vi "ArmControlManual.vi"(5 "Override Height Limit":bool, 6 "Wrist PID?":bool, 7 "Extension Triggers":cluster{"Retract":dbl, "Extend":dbl}, 8 "error in (no error)":errorcluster, 9 "Pivot Stick":cluster{"X":dbl, "Y":dbl}, 10 "Wrist Stick":cluster{"X":dbl, "Y":dbl}, 11 "Pivot Multiplier":dbl=0.75) -> (0 "error out":errorcluster)   [LabVIEW 2015]
uses:
  <vilib>/Rock Robotics/WPI/CAN/TalonSRX/WPI_CANTalonSRX_APIControlMode.ctl
  Robot Global Data.vi
panel:
  in  "Retract Multiplier":dbl=0.6
  in  "Wrist Multiplier":dbl=45.0 format="%#_13g"
  in  "Extend Multiplier":dbl=1.0
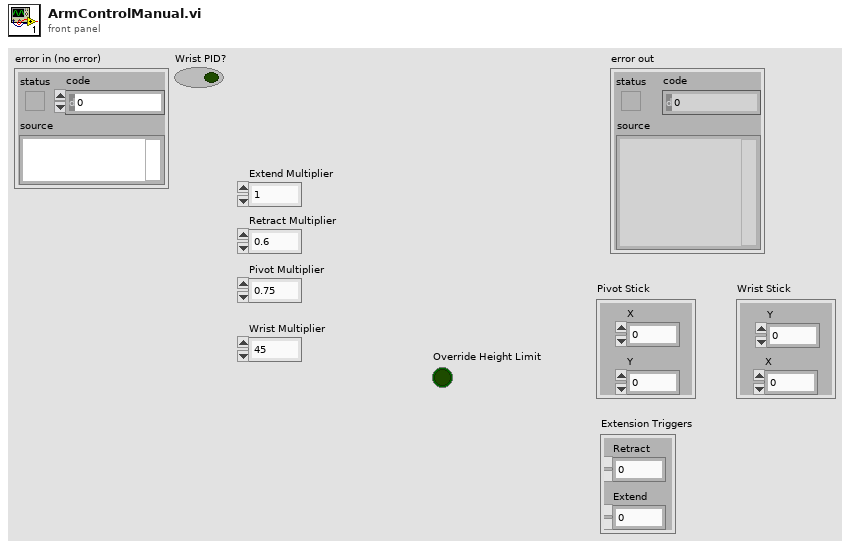
[diagram p1: front panel]
types:
  T1 = typedef "WPI_MotorControlDeviceRef.ctl" = cluster{"DeviceStatus":errorcluster, "Type":T2, "PWM":cluster{"PWM Channel":T3, "DeadBand":T4}, "CAN":cluster{"Device Number":u8, "Control Mode":T5, "Semaphore":T6, "Max Vout":dbl, "TalonSRX Control Mode":T7}, "Invert":bool, "TransformRef":T8, "InvTransformRef":T8}
  T2 = typedef "WPI_MotorControlType.ctl" = enum16{"PWM", "CAN", "CANTalonSRX"}
  T3 = typedef "FPGA_DIOPWMChannel.ctl" = enum8{"PWM 0", "PWM 1", "PWM 2", "PWM 3", "PWM 4", "PWM 5", "PWM 6", "PWM 7", "PWM 8", "PWM 9", "PWM MXP 0", "PWM MXP 1", "PWM MXP 2", "PWM MXP 3", "PWM MXP 4", "PWM MXP 5", "PWM MXP 6", "PWM MXP 7", "PWM MXP 8", "PWM MXP 9", "Invalid"}
  T4 = typedef "WPI_PWMDeadband.ctl" = cluster{"Name":string, "maxPositivePwm":i32, "minPositivePwm":i32, "centerPwm":i32, "maxNegativePwm":i32, "minNegativePwm":i32, "angularRange":u16}
  T5 = typedef "WPI_CANJaguar_ControlMode.ctl" = enum8{"Percent VBus", "Current", "Speed", "Position", "Voltage"}
  T6 = typedef "Semaphore RefNum" = refnum<k1>
  T7 = typedef "WPI_CANTalonSRX_APIControlMode.ctl" = enum8{"Percent VBus", "Speed", "Position", "Slave", "Unchanged / Invalid"}
  T8 = typedef "WPI_PWMTransform_ConPane.ctl" = refnum<vi>
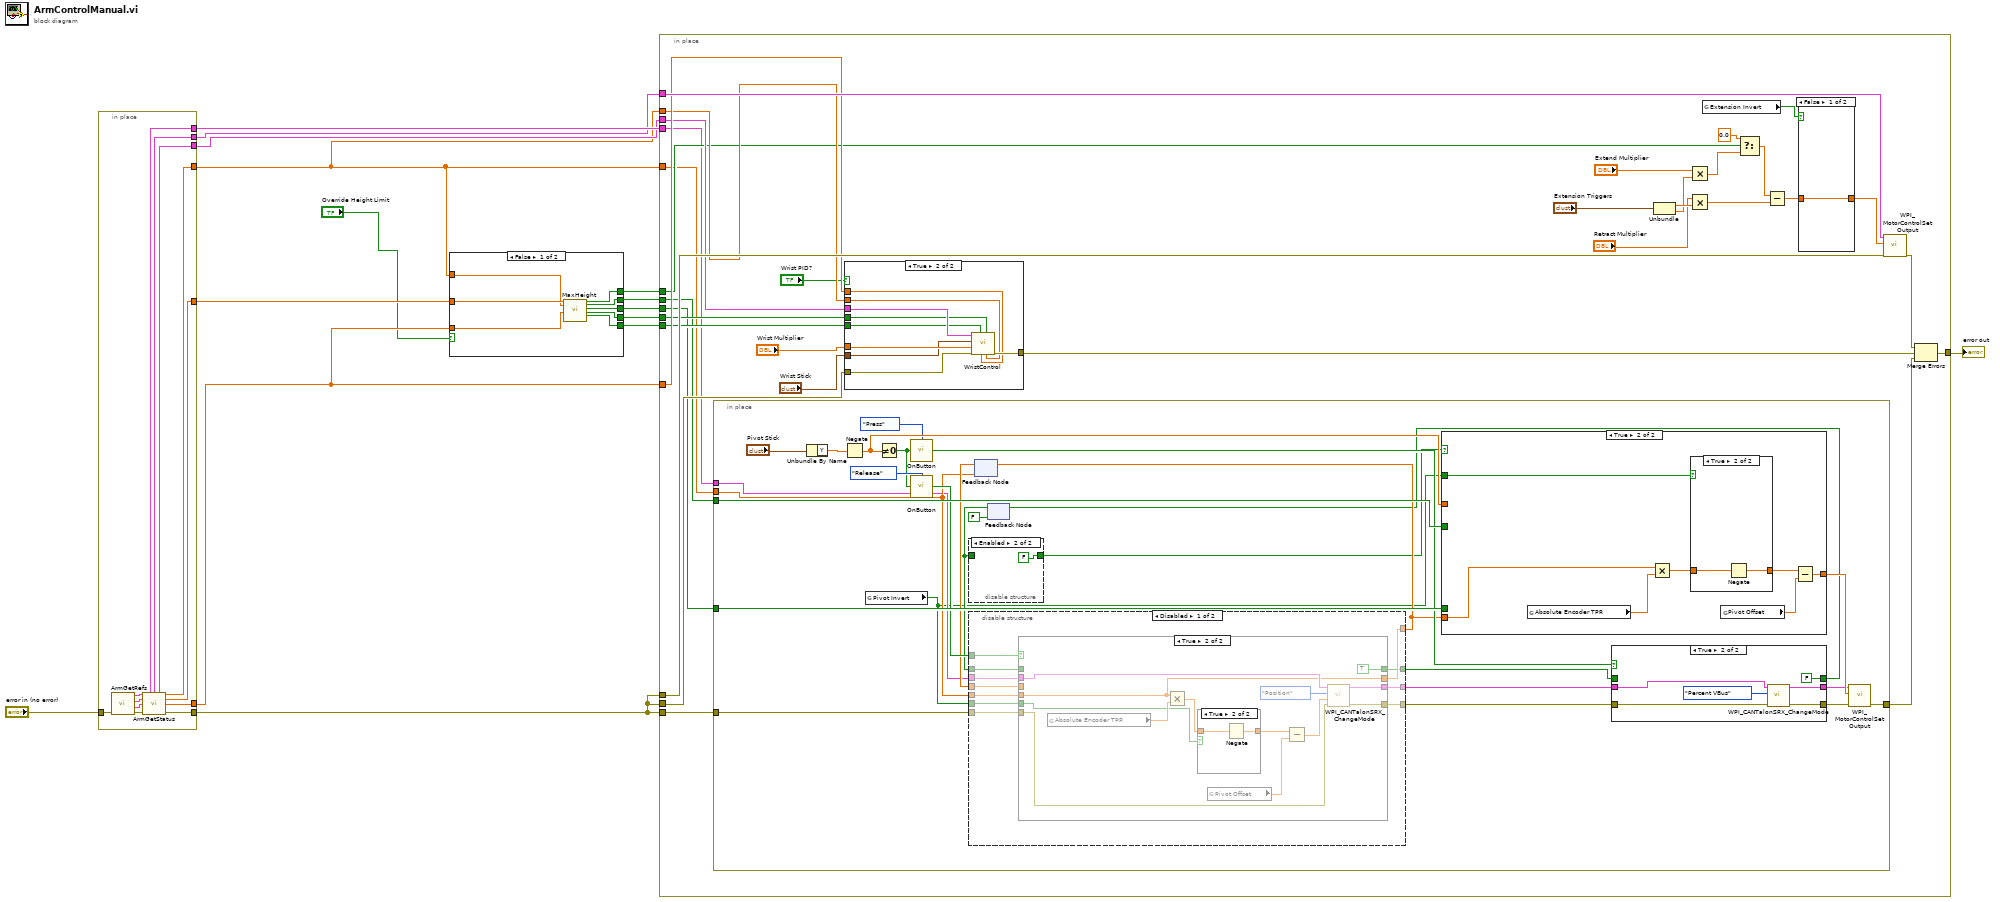
[diagram p0: block diagram]
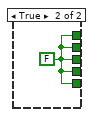
[diagram p2: hidden frame]
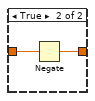
[diagram p3: hidden frame]
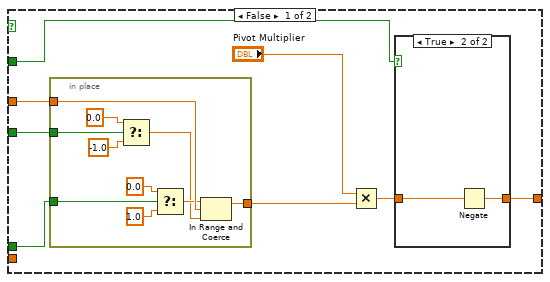
[diagram p9: hidden frame]
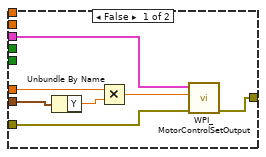
[diagram p12: hidden frame]
diagram:
  n1 = in-place {
    in-place-border: "error in (no error)" -> [w17]
    in-place-border: [w23] -> w14
    in-place-border: [w19] -> w10
    in-place-border: [w22] -> w8
    in-place-border: [w18] -> w12
    in-place-border: [w20] -> w2
    in-place-border: [w16] -> w11
    in-place-border: [w21] -> w9
    n2 = call "ArmGetRefs.vi"("error in (no error)"=w17) -> ("error out"=w24:errorcluster, "Wrist Ref"=w25:T1, "Extension Ref"=w26:T1, "Pivot Ref"=w27:T1)  [unwired: 7 in]
    n3 = call "ArmGetStatus.vi"("Pivot Ref"=w27, "ExtensionRef"=w26, "Wrist Ref"=w25, "error in (no error)"=w24) -> ("Pivot Ref out"=w18:T1, "Extension Ref out"=w19:T1, "Wrist Ref out"=w16:T1, "Pivot angle (rad)"=w20:dbl, "Extension (in.)"=w23:dbl, "Wrist angle (rad, relative to ground)"=w21:dbl, "error out"=w22:errorcluster)  [unwired: 3 in, 2 out]
  }
  n4 = case shown="False" "Override Height Limit" {
    tunnel: w14 -> [w35 _]
    tunnel: w9 -> [w34 _]
    tunnel: [w33 w36] -> w7
    tunnel: [w32 w36] -> w6
    tunnel: [w31 w36] -> w5
    tunnel: [w30 w36] -> w4
    tunnel: [w29 w36] -> w3
    tunnel: w2 -> [w28 _]
    frame False {
      n5 = call "MaxHeight.vi"("Extension Length"=w35, "Pivot Angle"=w28, "Wrist Angle (relative to ground)"=w34) -> ("Disable Extend"=w29:bool, "Disable Pivot Reverse"=w30:bool, "Disable Pivot Forward"=w31:bool, "Disable Wrist Reverse"=w33:bool, "Disable Wrist Forward"=w32:bool)  [unwired: 10 in, 2 out]
    }
    frame True {
      w36 = FALSE
    }
  }
  n6 = in-place {
    in-place-border: [w67] -> w15
    in-place-border: w12 -> [w39]
    in-place-border: w11 -> [w52]
    in-place-border: w10 -> [w61]
    in-place-border: w8 -> [w55]
    in-place-border: w9 -> [w54]
    in-place-border: w2 -> [w53]
    in-place-border: w8 -> [w51]
    in-place-border: w8 -> [w38]
    in-place-border: w7 -> [w45]
    in-place-border: w6 -> [w44]
    in-place-border: w5 -> [w43]
    in-place-border: w4 -> [w42]
    in-place-border: w3 -> [w41]
    in-place-border: w2 -> [w40]
    n7 = in-place {
      in-place-border: [w97] -> w65
      in-place-border: w43 -> [w95]
      in-place-border: w42 -> [w94]
      in-place-border: w40 -> [w89]
      in-place-border: w39 -> [w88]
      in-place-border: w38 -> [w87]
      n8 = Unbundle By Name("Pivot Stick") -> ("Y"=w96:dbl)
      n9 = Negate(x=w96) -> (-x=w93:dbl)
      n10 = global read "Robot Global Data.vi" "Pivot Invert"() -> (w73:bool)
      n11 = Not Equal To 0?(x=w93) -> (x != 0?=w85:bool)
      n12 = call "OnButton.vi"("Button"=w85, "Mode"=enum16{"Press", "Release", "Both"}."Press") -> ("Value"=w84:bool)
      n13 = call "OnButton.vi"("Button"=w85, "Mode"=enum16{"Press", "Release", "Both"}."Release") -> ("Value"=w91:bool)
      n14 = feedback #1(w89) -> (w90:dbl)
      n15 = feedback #2(FALSE) -> (w74:bool)
      n16 = disable-structure shown="Enabled" {
        disable-tunnel: [w100 FALSE] -> w75
        disable-tunnel: w74 -> [w100 _]
        frame Disabled {
        }
        frame Enabled {
        }
      }
      n17 = disable-structure shown="Disabled" {
        disable-tunnel: w91 -> [w112 _]
        disable-tunnel: w90 -> [w111 _]
        disable-tunnel: w89 -> [w110 _]
        disable-tunnel: w88 -> [w109 w134]
        disable-tunnel: w87 -> [w108 w133]
        disable-tunnel: [w107 w134] -> w83
        disable-tunnel: [w106 w133] -> w82
        disable-tunnel: [w105 _] -> w79
        disable-tunnel: [w104 _] -> w78
        disable-tunnel: w74 -> [w103 _]
        disable-tunnel: w73 -> [w102 _]
        frame Disabled {
          n18 = case shown="True" w112 {
            tunnel: w110 -> [_ w121]
            tunnel: [w114 w121] -> w105
            tunnel: w111 -> [w114 _]
            tunnel: w109 -> [w116 w129]
            tunnel: w108 -> [w115 w128]
            tunnel: [w115 w127] -> w106
            tunnel: [w116 w126] -> w107
            tunnel: [w113 TRUE] -> w104
            tunnel: w103 -> [w113 _]
            tunnel: w102 -> [_ w117]
            frame False {
            }
            frame True {
              n19 = global read "Robot Global Data.vi" "Absolute Encoder TPR"() -> (w123:dbl)
              n20 = Multiply(x=w121, y=w123) -> (x*y=w119:dbl)
              n21 = case shown="True" w117 {
                tunnel: w119 -> [w130 w132]
                tunnel: [w130 w131] -> w118
                frame False {
                }
                frame True {
                  n22 = Negate(x=w132) -> (-x=w131:dbl)
                }
              }
              n23 = global read "Robot Global Data.vi" "Pivot Offset"() -> (w122:dbl)
              n24 = Subtract(x=w118, y=w122) -> (x-y=w120:dbl)
              n25 = call <vilib>:"WPI_CANTalonSRX_ChangeMode.vi"("error in (no error)"=w128, "Output"=w120, "Control Mode"=WPI_CANTalonSRX_APIControlMode."Position", "CAN Talon SRX Ref"=w129) -> ("error out"=w127:errorcluster, "CAN Talon SRX Ref"=w126:T1)  [unwired: 6 in]
            }
          }
        }
        frame Enabled {
        }
      }
      n26 = feedback-in #1(w79) -> ()
      n27 = case shown="True" w75 {
        tunnel: [w144 w168] -> w98
        tunnel: w95 -> [w149 _]
        tunnel: w94 -> [w148 _]
        tunnel: w93 -> [w147 _]
        tunnel: w79 -> [_ w170]
        tunnel: w73 -> [w146 w165]
        frame False {
          n28 = in-place {
            in-place-border: w147 -> [w164]
            in-place-border: [w161] -> w150
            in-place-border: w149 -> [w156]
            in-place-border: w148 -> [w155]
            n29 = Select(t=0.0, s=w155, f=-1.0) -> (s? t:f=w162:dbl)
            n30 = Select(t=0.0, s=w156, f=1.0) -> (s? t:f=w163:dbl)
            n31 = In Range and Coerce(upper limit=w163, x=w164, lower limit=w162) -> (coerced(x)=w161:dbl)  [unwired: 1 out]
          }
          n32 = Multiply(x="Pivot Multiplier", y=w150) -> (x*y=w145:dbl)
          n33 = case shown="True" w146 {
            tunnel: w145 -> [w152 w154]
            tunnel: [w152 w153] -> w144
            frame False {
            }
            frame True {
              n34 = Negate(x=w154) -> (-x=w153:dbl)
            }
          }
        }
        frame True {
          n35 = global read "Robot Global Data.vi" "Absolute Encoder TPR"() -> (w171:dbl)
          n36 = Multiply(x=w170, y=w171) -> (x*y=w169:dbl)
          n37 = case shown="True" w165 {
            tunnel: w169 -> [w172 w174]
            tunnel: [w172 w173] -> w166
            frame False {
            }
            frame True {
              n38 = Negate(x=w174) -> (-x=w173:dbl)
            }
          }
          n39 = global read "Robot Global Data.vi" "Pivot Offset"() -> (w167:dbl)
          n40 = Subtract(x=w166, y=w167) -> (x-y=w168:dbl)
        }
      }
      n41 = case shown="True" w84 {
        tunnel: w83 -> [w137 w143]
        tunnel: w82 -> [w136 w142]
        tunnel: [w136 w141] -> w81
        tunnel: [w137 w140] -> w80
        tunnel: w78 -> [w135 _]
        tunnel: [w135 FALSE] -> w77
        frame False {
        }
        frame True {
          n42 = call <vilib>:"WPI_CANTalonSRX_ChangeMode.vi"("error in (no error)"=w142, "Control Mode"=WPI_CANTalonSRX_APIControlMode."Percent VBus", "CAN Talon SRX Ref"=w143) -> ("error out"=w141:errorcluster, "CAN Talon SRX Ref"=w140:T1)  [unwired: 7 in]
        }
      }
      n43 = feedback-in #2(w77) -> ()
      n44 = call <vilib>:"WPI_MotorControlSetOutput.vi"("error in (no error)"=w81, "Output"=w98, "MotorControlDevRef"=w80) -> ("error out"=w97:errorcluster)  [unwired: 6 in, 2 out]
    }
    n45 = case shown="True" "Wrist PID?" {
      tunnel: w54 -> [_ w186]
      tunnel: w53 -> [_ w185]
      tunnel: w52 -> [w180 w188]
      tunnel: [w177 w189] -> w48
      tunnel: w51 -> [w178 w190]
      tunnel: "Wrist Multiplier" -> [w181 w187]
      tunnel: "Wrist Stick" -> [w176 w184]
      tunnel: w45 -> [_ w183]
      tunnel: w44 -> [_ w182]
      frame False {
        n46 = Unbundle By Name(w176) -> ("Y"=w175:dbl)
        n47 = Multiply(x=w181, y=w175) -> (x*y=w179:dbl)
        n48 = call <vilib>:"WPI_MotorControlSetOutput.vi"("error in (no error)"=w178, "Output"=w179, "MotorControlDevRef"=w180) -> ("error out"=w177:errorcluster)  [unwired: 6 in, 2 out]
      }
      frame True {
        n49 = call "WristControl.vi"("Pivot Angle"=w185, "Disable Wrist Forward"=w183, "Wrist Angle (relative to ground)"=w186, "Disable Wrist Back"=w182, "error in (no error)"=w190, "Wrist Multiplier (degrees/second)"=w187, "Wrist Stick"=w184, "MotorControlDevRef"=w188) -> ("error out"=w189:errorcluster)  [unwired: 1 in, 2 out]
      }
    }
    n50 = Unbundle("Extension Triggers") -> ("Retract"=w63:dbl, "Extend"=w59:dbl)
    n51 = Multiply(x="Extend Multiplier", y=w59) -> (x*y=w58:dbl)
    n52 = Multiply(x="Retract Multiplier", y=w63) -> (x*y=w57:dbl)
    n53 = global read "Robot Global Data.vi" "Extension Invert"() -> (w37:bool)
    n54 = Select(t=0.0, s=w41, f=w58) -> (s? t:f=w64:dbl)
    n55 = Subtract(x=w64, y=w57) -> (x-y=w60:dbl)
    n56 = case shown="False" w37 {
      tunnel: w60 -> [w70 w72]
      tunnel: [w70 w71] -> w46
      frame False {
      }
      frame True {
        n57 = Negate(x=w72) -> (-x=w71:dbl)
      }
    }
    n58 = call <vilib>:"WPI_MotorControlSetOutput.vi"("error in (no error)"=w55, "Output"=w46, "MotorControlDevRef"=w61) -> ("error out"=w66:errorcluster)  [unwired: 6 in, 2 out]
    n59 = Merge Errors(w66, w48, w65) -> (w67:errorcluster)
  }
  "error out" <- w15
